vi "Format Blob Service Properties.vi"(11 "Blob service properties":T1) -> (3 "Blob service string":string)   [LabVIEW 2015, in "NI_Azure_Blob.lvlib"]
uses:
  NI_Azure_Blob.lvlib
  Blob Service Properties.ctl
  Logging.ctl
  Retention Policy.ctl
  Metrics.ctl
  Cors Rule.ctl
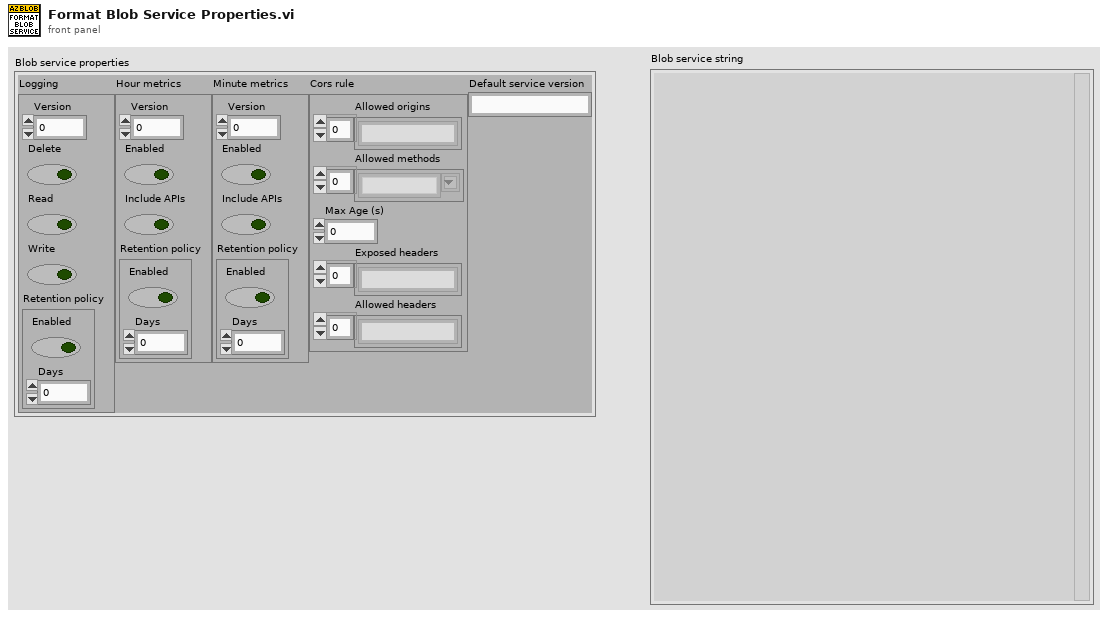
[diagram p1: front panel]
types:
  T1 = typedef "NI_Azure_Blob.lvlib/Blob Service Properties.ctl" = cluster{"Logging":T2, "Hour metrics":T4, "Minute metrics":T4, "Cors rule":T5, "Default service version":string}
  T2 = typedef "NI_Azure_Blob.lvlib/Logging.ctl" = cluster{"Version":dbl, "Delete":bool, "Read":bool, "Write":bool, "Retention policy":T3}
  T3 = typedef "NI_Azure_Blob.lvlib/Retention Policy.ctl" = cluster{"Enabled":bool, "Days":u32}
  T4 = typedef "NI_Azure_Blob.lvlib/Metrics.ctl" = cluster{"Version":dbl, "Enabled":bool, "Include APIs":bool, "Retention policy":T3}
  T5 = typedef "NI_Azure_Blob.lvlib/Cors Rule.ctl" = cluster{"Allowed origins":string[], "Allowed methods":string[], "Max Age (s)":u32, "Exposed headers":string[], "Allowed headers":string[]}
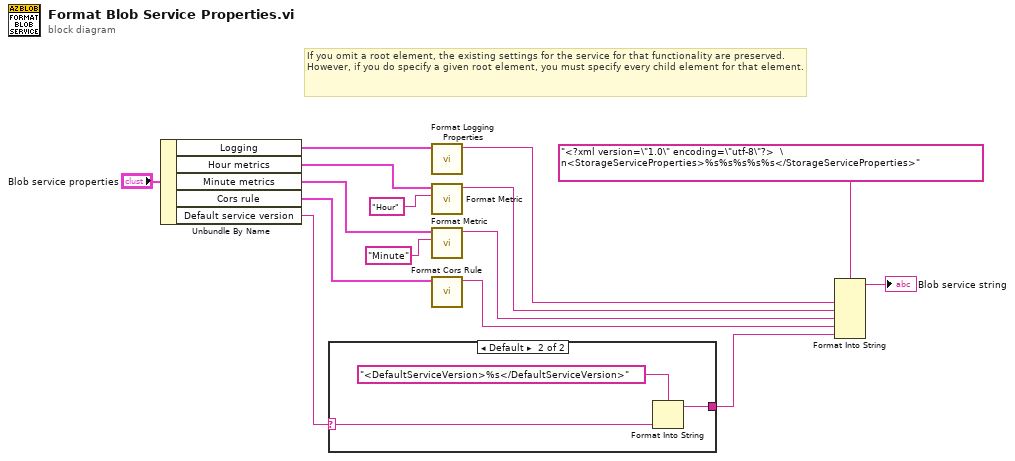
[diagram p0: block diagram]
diagram:
  # "If you omit a root element, the existing settings for the service for that functionality are preserved. However, if you do specify a given root element, you must specify every child element for that element."
  n1 = Unbundle By Name("Blob service properties") -> ("Logging"=w14:T2, "Hour metrics"=w11:T4, "Minute metrics"=w10:T4, "Cors rule"=w4:T5, "Default service version"=w1:string)
  n2 = case shown="Default" w1 {
    selector: w1 -> [_ w16]
    tunnel: [_ w17] -> w2
    frame "" {
    }
    frame Default {
      n3 = Format Into String(format string="<DefaultServiceVersion>%s</DefaultServiceVersion>", w16) -> (resulting string=w17:string)  [unwired: 2 in, 1 out]
    }
  }
  n4 = call "Format Logging Properties.vi"("Logging properties"=w14) -> ("Logging string"=w8:string)  [unwired: 10 in]
  n5 = call "Format Metric.vi"("Metric name"="Hour", "Metric properties"=w11) -> ("Metrics string"=w7:string)  [unwired: 9 in]
  n6 = call "Format Metric.vi"("Metric name"="Minute", "Metric properties"=w10) -> ("Metrics string"=w6:string)  [unwired: 9 in]
  n7 = call "Format Cors Rule.vi"("Cors rule"=w4) -> ("Cors rule string"=w3:string)  [unwired: 10 in]
  n8 = Format Into String(format string="<?xml version=\"1.0\" encoding=\"utf-8\"?>  \n<StorageServiceProperties>%s%s%s%s%s</StorageServiceProperties>", w8, w7, w6, w3, w2) -> (resulting string=→"Blob service string":string)  [unwired: 2 in, 1 out]
